vi "Create Calibers table from Server DB.vi"(8 "error in":errorcluster) -> (0 "error out":errorcluster)   [LabVIEW 2010]
uses:
  <vilib>/addons/database/NI_Database_API.lvlib
  <vilib>/addons/database/Connection.llb/DB Tools Open Connec (Path).vi
  <vilib>/addons/database/Connection.llb/Conn Execute.vi
  <vilib>/addons/database/Recordset.llb/Rec Fetch Recordset Data (R).vi
  <vilib>/addons/database/Auxilliary.llb/DB Tools Cursor Type.ctl
  <vilib>/addons/database/Recordset.llb/Rec Destroy - Connection.vi
  <vilib>/addons/database/_DB Variant To Data/Database Variant To Data.xnode
  <vilib>/addons/database/Auxilliary.llb/DB Tools DataTypes.ctl
panel:
  in  "Table":string="ThreatCalibers"
  out "column information":T2(array[cluster])
  out "columns":string[](array[string])
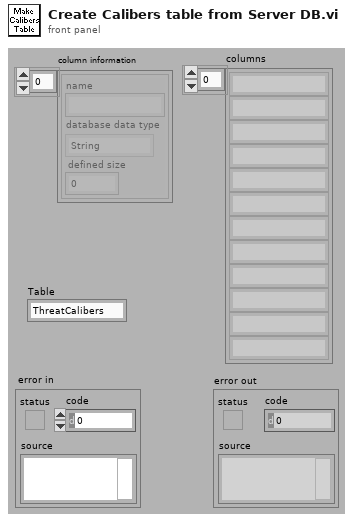
[diagram p1: front panel]
types:
  T1 = typedef "NI_Database_API.lvlib/DB Tools DataTypes.ctl" = enum16{"String", "Long (I32)", "Single (SGL)", "Double (DBL)", "Date/Time", "Binary"}
  T2 = cluster{"name":string, "database data type":T1, "defined size":i32}[]
  T3 = typedef "NI_Database_API.lvlib/DB Tools Cursor Type.ctl" = enum16{"forward-only", "keyset", "dynamic", "static"}
  T4 = typedef "NI_Database_API.lvlib/Conn ObjectReference.ctl" = refnum<k1>
  T5 = typedef "NI_Database_API.lvlib/Rec ObjectReference.ctl" = refnum<k1>
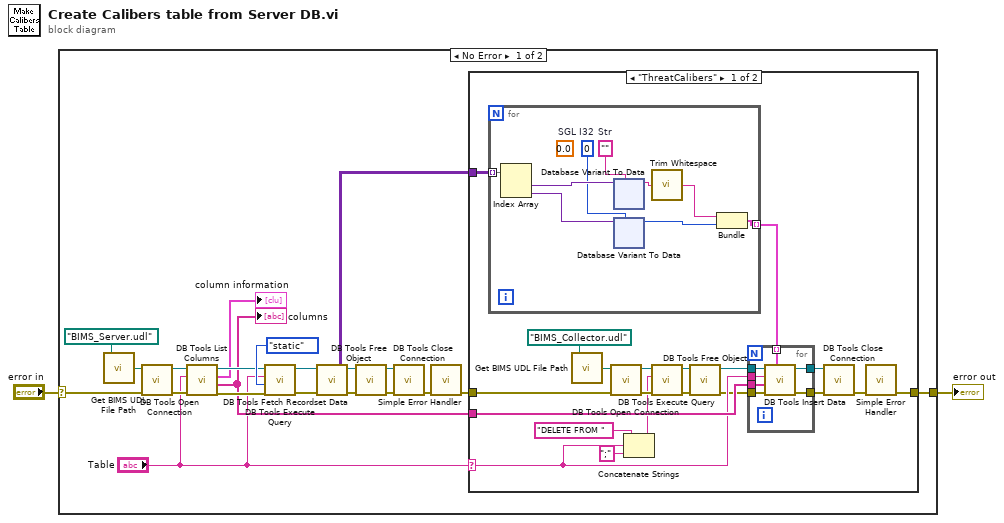
[diagram p0: block diagram]
diagram:
  n1 = case shown="No Error" "error in" {
    selector: "error in" -> [w3 w125]
    tunnel: [w4 w125] -> w2
    frame No Error {
      n2 = call "Get BIMS UDL File Path.vi"("UDL file name"=path "BIMS_Server.udl") -> ("Full UDL file path"=w22:path)
      n3 = call-poly <vilib>:"DB Tools Open Connection.vi"("error in (no error)"=w3, "connection information"=w22) -> ("error out"=w20:errorcluster, "connection reference"=w21:T4)  [unwired: 3 in, 3 out]
      n4 = call <vilib>:"DB Tools List Columns.vi"("error in (no error)"=w20, "table"="Table", "connection reference"=w21) -> ("error out"=w9:errorcluster, "columns"=w6:string[], "column information"=→"column information":T2, "connection reference out"=w10:T4)  [unwired: 1 out]
      "columns" <- w6
      n5 = call-poly <vilib>:"DB Tools Execute Query.vi"("error in (no error)"=w9, "cursor type"=DB_Tools_Cursor_Type."static", "SQL query"="Table", "connection reference"=w10) -> ("error out"=w13:errorcluster, "recordset reference"=w14:T5)  [unwired: 4 out]
      n6 = call-poly <vilib>:"DB Tools Fetch Recordset Data.vi"("error in (no error)"=w13, "recordset reference"=w14) -> ("error out"=w16:errorcluster, "recordset data"=w11:variant[][], "recordset reference out"=w15:T5)  [unwired: 3 out]
      n7 = call-poly <vilib>:"DB Tools Free Object.vi"("error in (no error)"=w16, "recordset reference"=w15) -> ("error out"=w18:errorcluster, "connection reference"=w17:T4)  [unwired: 8 out]
      n8 = call <vilib>:"DB Tools Close Connection.vi"("error in (no error)"=w18, "connection reference"=w17) -> ("error out"=w8:errorcluster)  [unwired: 5 out]
      n9 = call <vilib>:"Simple Error Handler.vi"("error in (no error)"=w8) -> ("error out"=w19:errorcluster)  [unwired: 1 in, 7 out]
      n10 = case shown="\"ThreatCalibers\"" "Table" {
        selector: "Table" -> [w30 _]
        tunnel: w19 -> [w43 w124]
        tunnel: w11 -> [w42 _]
        tunnel: w6 -> [w38 _]
        tunnel: [w34 w124] -> w4
        frame "ThreatCalibers" {
          n11 = for {
            tunnel: [w55] -> w35 mode=indexing
            tunnel: w42 -> [w59] mode=indexing
            (unwired) sgl 0.0  # SGL
            w51 = ""  # Str
            w52 = 0  # I32
            n12 = Index Array(array=w59) -> (element #1=w58:variant, element #2=w57:variant)  [unwired: 2 in]
            n13 = xnode ("Database Variant To Data")("database variant"=w58, "type"=w51) -> ("data"=w54:string)  [unwired: 1 in, 1 out]
            n14 = xnode "Database Variant To Data"("database variant"=w57, "type"=w52) -> ("data"=w56:i32)  [unwired: 1 in, 1 out]
            n15 = call <vilib>:"Trim Whitespace.vi"("string"=w54) -> ("trimmed string"=w53:string)  [unwired: 1 in]
            n16 = Bundle("trimmed string"=w53, "data"=w56) -> (w55:cluster{"trimmed string":string, "data":i32})  [unwired: 1 out]
          }
          n17 = call "Get BIMS UDL File Path.vi"("UDL file name"=path "BIMS_Collector.udl") -> ("Full UDL file path"=w41:path)
          n18 = call-poly <vilib>:"DB Tools Open Connection.vi"("error in (no error)"=w43, "connection information"=w41) -> ("error out"=w33:errorcluster, "connection reference"=w29:T4)  [unwired: 3 in, 3 out]
          n19 = Concatenate Strings("DELETE FROM " ("SQL query"), w30, ";" ("string")) -> (w31:string)
          n20 = call-poly <vilib>:"DB Tools Execute Query.vi"("error in (no error)"=w33, "SQL query"=w31, "connection reference"=w29) -> ("error out"=w27:errorcluster, "recordset reference"=w25:T5)  [unwired: 1 in, 4 out]
          n21 = call-poly <vilib>:"DB Tools Free Object.vi"("error in (no error)"=w27, "recordset reference"=w25) -> ("error out"=w26:errorcluster, "connection reference"=w24:T4)  [unwired: 8 out]
          n22 = for {
            tunnel: [w50] -> w36
            tunnel: [w46] -> w37
            tunnel: w26 -> [w49]
            tunnel: w30 -> [w48]
            tunnel: w35 -> [w45] mode=indexing
            tunnel: w38 -> [w47]
            tunnel: w24 -> [w44]
            n23 = call <vilib>:"DB Tools Insert Data.vi"("data"=w45, "error in (no error)"=w49, "columns"=w47, "table"=w48, "connection reference"=w44) -> ("error out"=w46:errorcluster, "connection reference out"=w50:T4)  [unwired: 2 in, 3 out]
          }
          n24 = call <vilib>:"DB Tools Close Connection.vi"("error in (no error)"=w37, "connection reference"=w36) -> ("error out"=w40:errorcluster)  [unwired: 5 out]
          n25 = call <vilib>:"Simple Error Handler.vi"("error in (no error)"=w40) -> ("error out"=w34:errorcluster)  [unwired: 1 in, 7 out]
        }
        frame "Information", Default {
          # "The following case has a structure determined for \n  the Threats table in the BIMS server.\n\n  The data retieved from the table is site specific."
        }
      }
    }
    frame Error {
    }
  }
  "error out" <- w2
